vi "Untitled 9.vi"() -> ()   [LabVIEW 2016, in "System.lvlib"]
uses:
  System.lvlib
panel:
  in  "Error":refnum<user-event>
  in  "Stop":refnum<user-event>
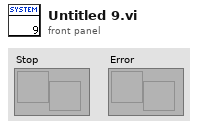
[diagram p1: front panel]
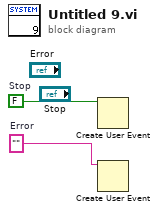
[diagram p0: block diagram]
diagram:
  w1 = ""  # Error
  w2 = FALSE  # Stop
  n1 = Create User Event(user event datatype=w2) -> ()  [unwired: 1 in, 2 out]
  n2 = Create User Event(user event datatype=w1) -> ()  [unwired: 1 in, 2 out]
